vi "WriteDO.vi"(8 "error in":errorcluster, 9 "DO Value":bool, 10 "Output":T1, 11 "VISA resource name":refnum<visa-resource-name>) -> (0 "error out":errorcluster, 3 "VISA resource name out":refnum<visa-resource-name>)   [LabVIEW 2020, in "HandsOnPi2040.lvlib"]
doc: "Establishes communication with the instrument and optionally performs an instrument identification query and/or an instrument reset. It also places the instrument in a default state needed for other instrument driver operations. Therefore, call this VI before calling other instrument driver VIs for this instrument. Generally, you need to call the <b>Initialize</b> VI only once at the beginning of an application."
uses:
  HandsOnPi2040.lvlib
  DigOuts.ctl
  <vilib>/CTI/CTI Visa Drivers/CTI-Visa/CTI-Visa.lvlib
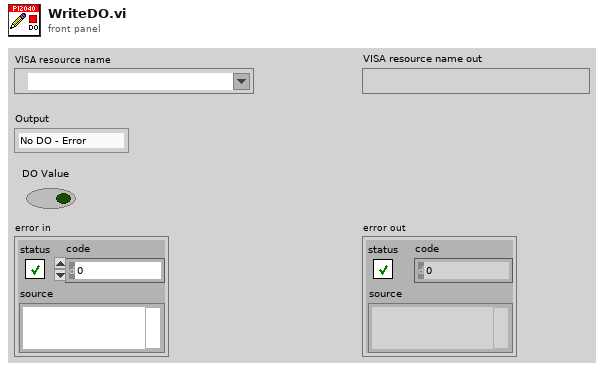
[diagram p1: front panel]
types:
  T1 = typedef "HandsOnPi2040.lvlib/DigOuts.ctl" = enum16{"No DO - Error", "DO1 (GPIO2)", "DO2 (GPIO3)", "DO3 (GPIO4)", "DO4 (GPIO5)", "BEEP (GPIO6)"}
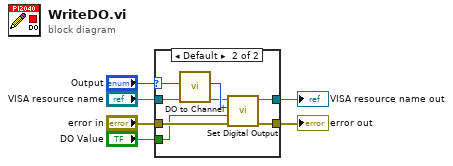
[diagram p0: block diagram]
diagram:
  n1 = case shown="Default" "Output" {
    selector: "Output" -> [_ w9]
    tunnel: [w8 w14] -> w5
    tunnel: [w7 w12] -> w4
    tunnel: "VISA resource name" -> [w7 w11]
    tunnel: "error in" -> [w8 w15]
    tunnel: "DO Value" -> [_ w10]
    frame "No DO - Error" {
    }
    frame Default {
      n2 = call "DO to Channel.vi"("Output"=w9) -> ("Channel"=w13:i32)  [unwired: 10 in]
      n3 = call <vilib>:"Set Digital Output.vi"("error in (no error)"=w15, "Value"=w10, "Channel"=w13, "VISA resource name in"=w11) -> ("error out"=w14:errorcluster, "VISA resource name"=w12:refnum<visa-resource-name>)  [unwired: 6 in]
    }
  }
  "VISA resource name out" <- w4
  "error out" <- w5
